vi "getDebugMode.vi"() -> (3 "debugMode":bool)   [LabVIEW 2011]
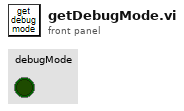
[diagram p1: front panel]
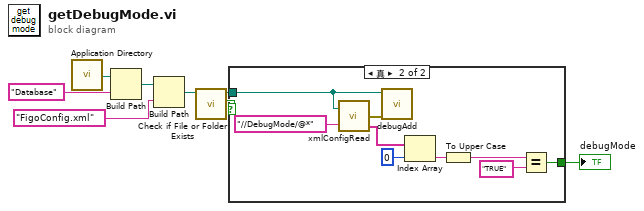
[diagram p0: block diagram]
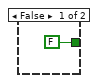
[diagram p2: hidden frame]
diagram:
  n1 = call <vilib>:"Application Directory.vi"() -> ("Application Directory"=w6:path)
  n2 = Build Path(base path=w6, name or relative path="Database" ("名称或相对路径")) -> (appended path=w8:path)
  n3 = Build Path(base path=w8, name or relative path="FigoConfig.xml" ("名称或相对路径")) -> (appended path=w5:path)
  n4 = call <vilib>:"Check if File or Folder Exists.vi"("path"=w5) -> ("file or folder exists?"=w4:bool, "dup path"=w3:path)  [unwired: 8 in, 1 out]
  n5 = case shown="真" w4 {
    tunnel: w3 -> [_ w11]
    tunnel: [FALSE w15] -> w1
    frame False {
    }
    frame True {
      n6 = call "xmlConfigRead.vi"("path to XML document"=w11, "XPath expression"="//DebugMode/@*") -> ("error out"=w10:errorcluster, "OutParaArray"=w14:string[])  [unwired: 1 out]
      n7 = call "debugAdd.vi"("error in (no error)"=w10, "xmlConfigPath"=w11) -> ()  [unwired: 9 in, 1 out]
      n8 = Index Array(array=w14, index=0 ("索引")) -> (element=w12:string)
      n9 = To Upper Case(1:w12) -> (0:w17:string)
      n10 = Equal?(x=w17, y="TRUE") -> (x = y?=w15:bool)
    }
  }
  "debugMode" <- w1
